vi "使用循环构造数组.vi"() -> ()   [LabVIEW 2020]
panel:
  out "while循环构造数组":dbl[](array[numeric])
  out "for循环构造数组":dbl[](array[numeric])
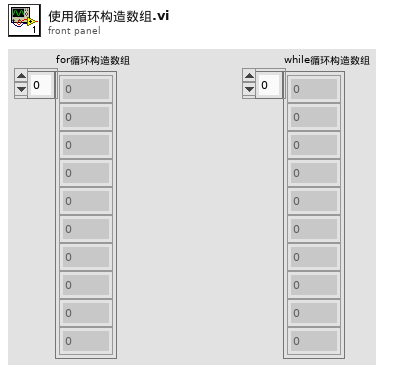
[diagram p1: front panel]
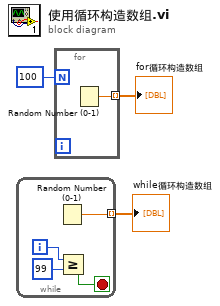
[diagram p0: block diagram]
diagram:
  n1 = while {
    tunnel: [w7] -> w1 mode=indexing
    i -> [w6]
    stop <- w4 stop-if-true
    n2 = Random Number (0-1)() -> (number: 0 to 1=w7:dbl)
    n3 = Greater Or Equal?(x=w6, y=99) -> (x >= y?=w4:bool)
  }
  "while循环构造数组" <- w1
  n4 = for {
    N: 100 -> [_]
    tunnel: [w8] -> w2 mode=indexing
    n5 = Random Number (0-1)() -> (number: 0 to 1=w8:dbl)
  }
  "for循环构造数组" <- w2
